vi "tsdiag_can_report_DTC_by_status_mask.vi"(7 "DTC descriptor":T1={"DTC Byte Length"=3, "Status Byte Length"=1, "Add Data Byte Length"=0, "Byte Order"=enum."Motorola"}, 8 "error in (no error)":errorcluster, 9 "status mask":u8, 10 "ADiagModuleIndex":i32, 11 "path":path) -> (0 "error out":errorcluster, 1 "success?":bool, 2 "Return Type":i32, 3 "path out":path, 4 "status avail mask":u8, 5 "DTCs":T2(array[cluster]))   [LabVIEW 2014]
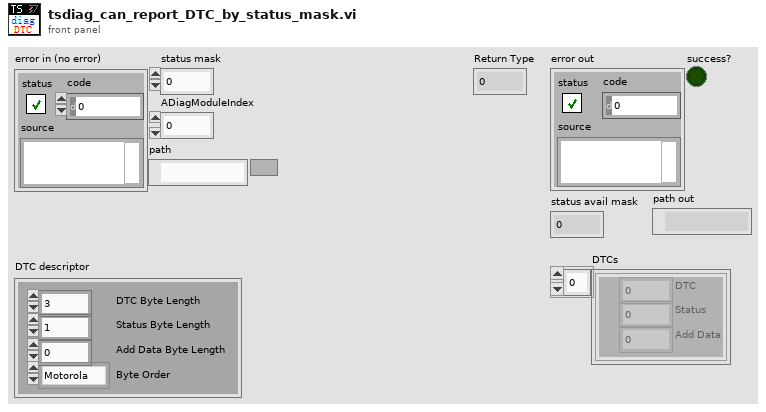
[diagram p1: front panel]
types:
  T1 = cluster{"DTC Byte Length":i32, "Status Byte Length":i32, "Add Data Byte Length":i32, "Byte Order":enum16{"Motorola", "Intel"}}
  T2 = cluster{"DTC":u32, "Status":u32, "Add Data":u32}[]
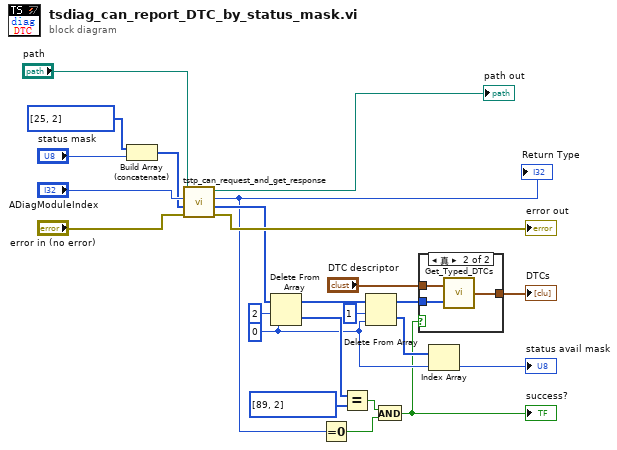
[diagram p0: block diagram]
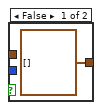
[diagram p2: hidden frame]
diagram:
  w12 = 0 ("index")
  n1 = Build Array (concatenate)(u8[] [25, 2], "status mask") -> (w4:u8[])
  n2 = call "tstp_can_request_and_get_response.vi"("错误输入（无错误）"="error in (no error)", "AReqDataArray"=w4, "ADiagModuleIndex"="ADiagModuleIndex", "path"="path") -> ("错误输出"=→"error out":errorcluster, "Diagnostic response"=w3:u8[], "Return Type"=w1:i32, "path out"=→"path out":path)  [unwired: 4 in]
  "Return Type" <- w1
  n3 = Delete From Array(array=w3, length=2, index=w12) -> (deleted portion=w23:u8[], array with subset deleted=w15:u8[])
  n4 = Equal To 0?(x=w1) -> (x = 0?=w2:bool)
  n5 = Equal?(x=w23, y=u8[] [89, 2]) -> (x = y?=w21:bool)
  n6 = Delete From Array(array=w15, length=1, index=w12) -> (deleted portion=w13:u8[], array with subset deleted=w14:u8[])
  n7 = And(x=w21, y=w2) -> (x .and. y?=w10:bool)
  "success?" <- w10
  n8 = case shown="真" w10 {
    tunnel: w14 -> [_ w28]
    tunnel: [T2 [] ("DTCs") w27] -> w20
    tunnel: "DTC descriptor" -> [_ w26]
    frame False {
    }
    frame True {
      n9 = call "Get_Typed_DTCs.vi"("data in"=w28, "DTC descriptor"=w26) -> ("DTCs"=w27:T2)
    }
  }
  "DTCs" <- w20
  n10 = Index Array(array=w13, index=w12) -> (element=→"status avail mask":u8)
